vi "Generate State Transition User Event.vi"(8 "error in (no error)":errorcluster, 11 "State Actor in":refnum<class "State Actor.lvclass">) -> (0 "error out":errorcluster, 3 "State Actor out":refnum<class "State Actor.lvclass">)   [LabVIEW 2024, in "State Actor.lvlib" / "State Actor.lvclass"]
uses:
  State Actor.lvclass
  State Transition Event.ctl
  State Actor.lvclass/State Actor.ctl
  C:/Program Files (x86)/National Instruments/LabVIEW 2024/vi.lib/ActorFramework/Actor/Actor.lvclass
  C:/Users/ottoa/OneDrive/Desktop/working copies/stateActor/src/State Actor/State Actor.lvclass
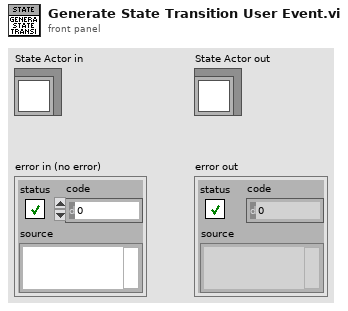
[diagram p1: front panel]
types:
  T1 = typedef "State Actor.lvlib/State Actor.lvclass/State Transition Event.ctl" = cluster{"Timestamp":timestamp, "State":string}
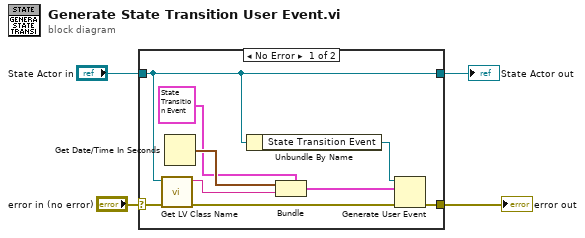
[diagram p0: block diagram]
diagram:
  n1 = case shown="No Error" "error in (no error)" {
    selector: "error in (no error)" -> [w6 w15]
    tunnel: [w12 w15] -> w3
    tunnel: [w8 w14] -> w1
    tunnel: "State Actor in" -> [w8 w14]
    frame No Error {
      n2 = call <vilib>:"Get LV Class Name.vi"("error in (no error)"=w6, "object"=w8) -> ("error out"=w5:errorcluster, "class name"=w7:string)  [unwired: 8 in]
      n3 = Get Date/Time In Seconds() -> (seconds since 1Jan1904=w11:timestamp)
      n4 = Unbundle By Name(w8) -> ("State Transition Event"=w13:refnum<user-event>)
      n5 = Bundle(cluster=T1 {"Timestamp"=timestamp(0 s since 1904-01-01), "State"=""} ("State Transition Event"), "Timestamp"=w11, "State"=w7) -> (w10:T1)
      n6 = Generate User Event(user event=w13, event data cluster=w10, error in=w5) -> (error out=w12:errorcluster)  [unwired: 1 in, 1 out]
    }
    frame Error {
    }
  }
  "error out" <- w3
  "State Actor out" <- w1
